vi "testTcpServer.vi"(8 "error in (no error)":errorcluster) -> (0 "error out":errorcluster)   [LabVIEW 2018]
doc: "Test TcpServer class."
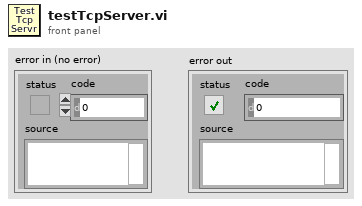
[diagram p1: front panel]
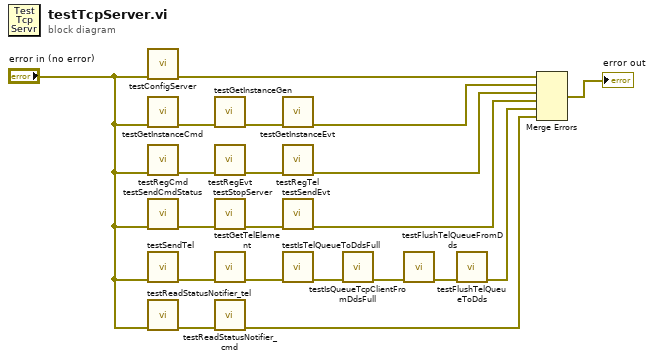
[diagram p0: block diagram]
diagram:
  n1 = call "testConfigServer.vi"("error in (no error)"="error in (no error)") -> ("error out"=w19:errorcluster)  [unwired: 10 in]
  n2 = call "testGetInstanceCmd.vi"("error in (no error)"="error in (no error)") -> ("error out"=w17:errorcluster)  [unwired: 10 in]
  n3 = call "testRegCmd.vi"("error in (no error)"="error in (no error)") -> ("error out"=w18:errorcluster)  [unwired: 10 in]
  n4 = call "testSendCmdStatus.vi"("error in (no error)"="error in (no error)") -> ("error out"=w14:errorcluster)  [unwired: 10 in]
  n5 = call "testSendTel.vi"("error in (no error)"="error in (no error)") -> ("error out"=w10:errorcluster)  [unwired: 10 in]
  n6 = call "testReadStatusNotifier_tel.vi"("error in (no error)"="error in (no error)") -> ("error out"=w2:errorcluster)  [unwired: 10 in]
  n7 = call "testGetInstanceGen.vi"("error in (no error)"=w17) -> ("error out"=w16:errorcluster)  [unwired: 10 in]
  n8 = call "testRegEvt.vi"("error in (no error)"=w18) -> ("error out"=w13:errorcluster)  [unwired: 10 in]
  n9 = call "testStopServer.vi"("error in (no error)"=w14) -> ("error out"=w12:errorcluster)  [unwired: 10 in]
  n10 = call "testGetTelElement.vi"("error in (no error)"=w10) -> ("error out"=w9:errorcluster)  [unwired: 10 in]
  n11 = call "testReadStatusNotifier_cmd.vi"("error in (no error)"=w2) -> ("error out"=w1:errorcluster)  [unwired: 10 in]
  n12 = call "testGetInstanceEvt.vi"("error in (no error)"=w16) -> ("error out"=w15:errorcluster)  [unwired: 10 in]
  n13 = call "testRegTel.vi"("error in (no error)"=w13) -> ("error out"=w6:errorcluster)  [unwired: 10 in]
  n14 = call "testSendEvt.vi"("error in (no error)"=w12) -> ("error out"=w11:errorcluster)  [unwired: 10 in]
  n15 = call "testIsTelQueueToDdsFull.vi"("error in (no error)"=w9) -> ("error out"=w8:errorcluster)  [unwired: 10 in]
  n16 = call "testIsQueueTcpClientFromDdsFull.vi"("error in (no error)"=w8) -> ("error out"=w4:errorcluster)  [unwired: 10 in]
  n17 = call "testFlushTelQueueFromDds.vi"("error in (no error)"=w4) -> ("error out"=w7:errorcluster)  [unwired: 10 in]
  n18 = call "testFlushTelQueueToDds.vi"("error in (no error)"=w7) -> ("error out"=w5:errorcluster)  [unwired: 10 in]
  n19 = Merge Errors(w19, w15, w6, w11, w5, w1) -> (→"error out":errorcluster)
